vi "MoveRel_all.vi"(7 "# axis":i32, 8 "error in (no error)":errorcluster, 10 "Position":dbl[](array[numeric]), 11 "VISA resource name":refnum<visa-resource-name>) -> (0 "error out":errorcluster)   [LabVIEW 2014, in "GRBLMotionCore.lvlib"]
doc: "Performs an instrument error query before terminating the software connection to the instrument."
uses:
  <instrlib>/GRBL/GRBLMotionCore.lvlib
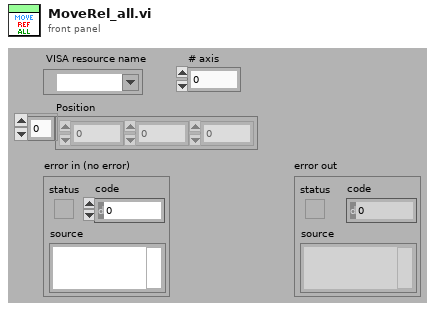
[diagram p1: front panel]
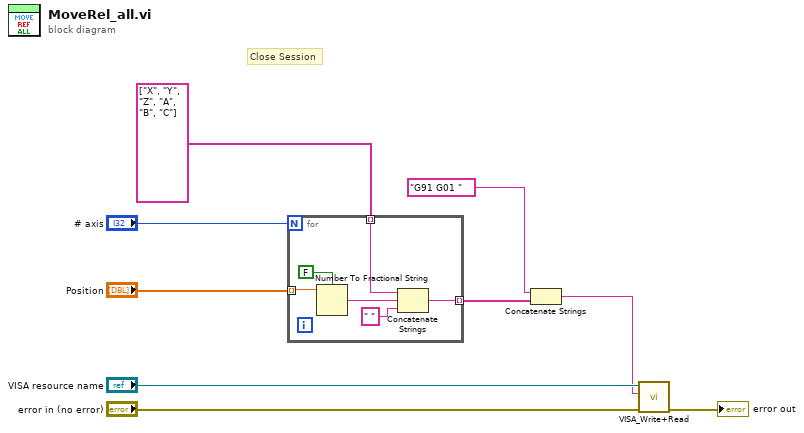
[diagram p0: block diagram]
diagram:
  # "Close Session"
  n1 = for {
    N: "# axis" -> [_]
    tunnel: "Position" -> [w15] mode=indexing
    tunnel: [w11] -> w6 mode=indexing
    tunnel: string[] ["X", "Y", "Z", "A", "B", "C"] -> [w10] mode=indexing
    n2 = Number To Fractional String(use system decimal point (T)=FALSE, number=w15) -> (F-format string=w13:string)  [unwired: 2 in]
    n3 = Concatenate Strings(w10, w13, " " ("string")) -> (w11:string)
  }
  n4 = Concatenate Strings("G91 G01 ", w6) -> (w3:string)
  n5 = call <instrlib>:"VISA_Write+Read.vi"("error in (no error)"="error in (no error)", "Write Buffer"=w3, "VISA resource name"="VISA resource name") -> ("error out"=→"error out":errorcluster)  [unwired: 6 in, 2 out]
